vi "ex_4c.vi"() -> ()   [LabVIEW 2020]
panel:
  out "Out 2":i32[][](array[numeric])
  out "Out 1":i32[][](array[numeric])
  out "Out 3":i32[][](array[numeric])
  in  "M":i32
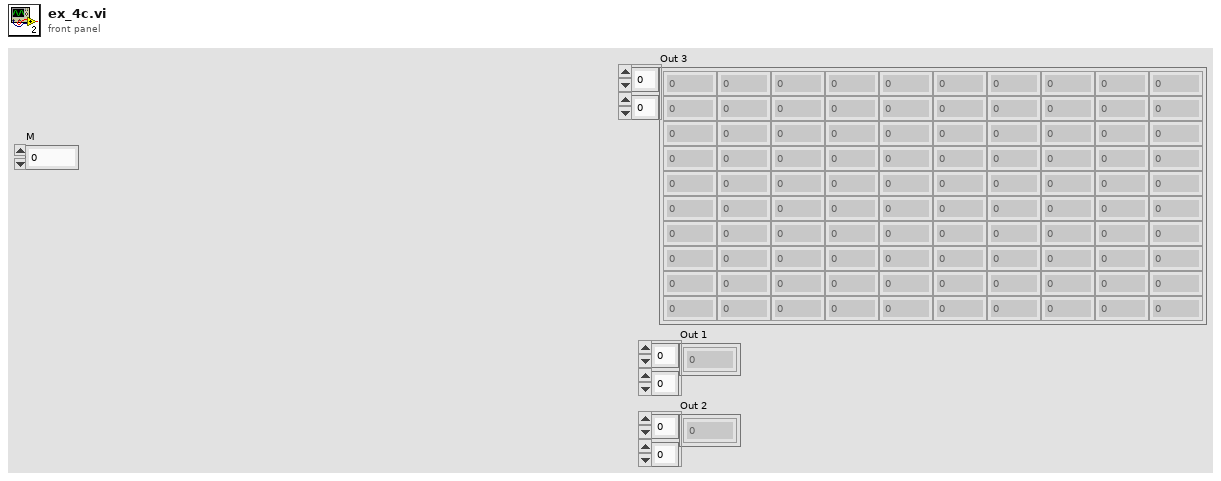
[diagram p1: front panel]
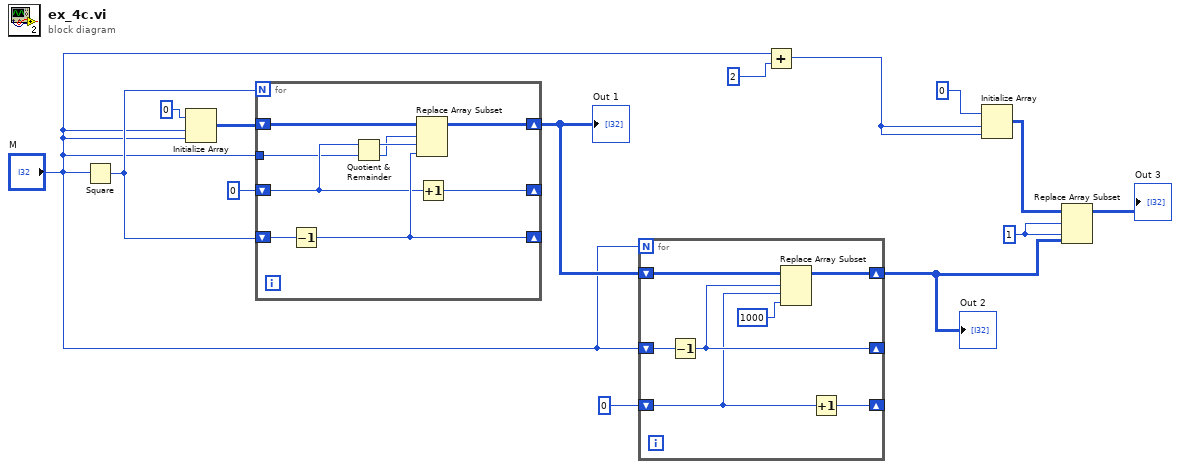
[diagram p0: block diagram]
diagram:
  w1 = 1 ("disabled index (col)")
  n1 = Square(x="M") -> (x^2=w14:i32)
  n2 = Initialize Array(0, "M", "M") -> (w12:i32[][])
  n3 = for {
    N: w14 -> [_]
    shift-right: [w21] -> w10
    shift-left: w12 -> [w23]
    shift-right: [w17] -> _
    shift-left: w14 -> [w22]
    shift-right: [w20] -> _
    shift-left: 0 -> [w16]
    tunnel: "M" -> [w15]
    n4 = Decrement(x=w22) -> (x-1=w17:i32)
    n5 = Quotient & Remainder(x=w16, y=w15) -> (x-y*floor(x/y)=w19:i32, floor(x/y)=w18:i32)
    n6 = Replace Array Subset(array=w23, new element=w17, index (row)=w18, index (col)=w19) -> (w21:i32[][])
    n7 = Increment(x=w16) -> (x+1=w20:i32)
  }
  "Out 1" <- w10
  n8 = for {
    N: "M" -> [_]
    shift-right: [w26] -> _
    shift-left: "M" -> [w30]
    shift-right: [w29] -> _
    shift-left: 0 -> [w25]
    shift-right: [w27] -> w3
    shift-left: w10 -> [w28]
    n9 = Decrement(x=w30) -> (x-1=w26:i32)
    n10 = Replace Array Subset(array=w28, new element=1000 ("new element/subarray"), index (row)=w26, index (col)=w25) -> (w27:i32[][])
    n11 = Increment(x=w25) -> (x+1=w29:i32)
  }
  "Out 2" <- w3
  n12 = Add(x="M", y=2 ("x")) -> (x+y=w8:i32)
  n13 = Initialize Array(0 ("element"), w8, w8) -> (w6:i32[][])
  n14 = Replace Array Subset(array=w6, new element=w3, index (row)=w1, index (col)=w1) -> (→"Out 3":i32[][])
